vi "Generate Parameter JSON (single).vi"(6 "Replace Empty with 'null'":bool=TRUE, 9 "Value in Quotes":bool=TRUE, 10 "Parameter Value":string, 11 "Parameter Name":string) -> (3 "Parameter JSON":string)   [LabVIEW 2015, in "NI_JSON Parsing.lvlib"]
uses:
  NI_JSON Parsing.lvlib
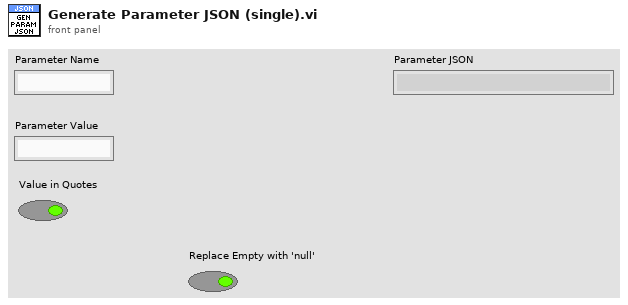
[diagram p1: front panel]
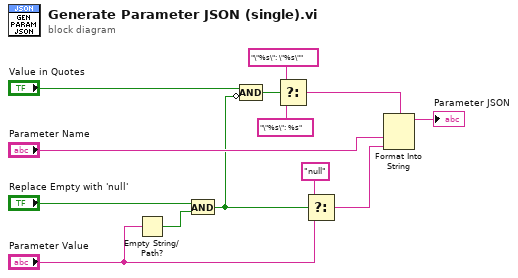
[diagram p0: block diagram]
diagram:
  n1 = Empty String/Path?(string/path="Parameter Value") -> (empty?=w3:bool)
  n2 = And(x="Replace Empty with 'null'", y=w3) -> (x .and. y?=w1:bool)
  n3 = Compound Arithmetic op=AND("Value in Quotes", invert w1) -> (w2:bool)
  n4 = Select(t="\"%s\": \"%s\"", s=w2, f="\"%s\": %s") -> (s? t:f=w10:string)
  n5 = Select(t="null", s=w1, f="Parameter Value") -> (s? t:f=w6:string)
  n6 = Format Into String(format string=w10, "Parameter Name", w6) -> (resulting string=→"Parameter JSON":string)  [unwired: 2 in, 1 out]
